vi "Trial data array-Initialise.vi"(6 "Total number of points in each \ntrial (or Z-plane), for both channels":u32, 8 "error in":errorcluster, 11 "Logging queue element":T1={"Imaging Protocol"=enum."Live Imaging", "Number of Trials"=0, "Frame Size"=512, "# Averaged frames"=0, "Dwell time (us)"=0.0, "Index of Z-plane"=0, "Timelapse?"=FALSE, "Logging process is active"=FALSE, "Speed logging enabled"=FALSE, "tdms file ref"=refnum, "path"=path "", "Trial Number"=0, "Expected # points acquired"=FALSE, "Manually stopped"=FALSE, "Last trial"=FALSE, "Ch0 data"=[], "Ch1 data"=[], "Ref Data"=[], "Ref Frame Time"=[], "Image Time"=[], "Continuous Time"=[], "Ref X Length"=0, "Ref Y Length"=0, "# Ref Averaged frames"=0, "Ref Dwell time (us)"=0.0, "Points acquired"={"Ch0 last trial"=0, "Ch1 last trial"=0, "All trials"=0}, "HW Timings File"=refnum} {"Ref Dwell time (us)" format="%#.6g"; "Frame Size" items=["100X100"=100, "128X128"=128, "200X200"=200, "256X256"=256, "512X512"=512, "1024x1024"=1024, "2048x2048"=2048]; "Dwell time (us)" format="%#.6g"}) -> (0 "error out":errorcluster, 1 "Initialised single trial or single plane data":dbl[](array[numeric]))   [LabVIEW 2020]
uses:
  Typedefs/Logging queue element.ctl
  Typedefs/Imaging Protocols enum.ctl
  Typedefs/Frame Size.ctl
  Typedefs/Acquired points count.ctl
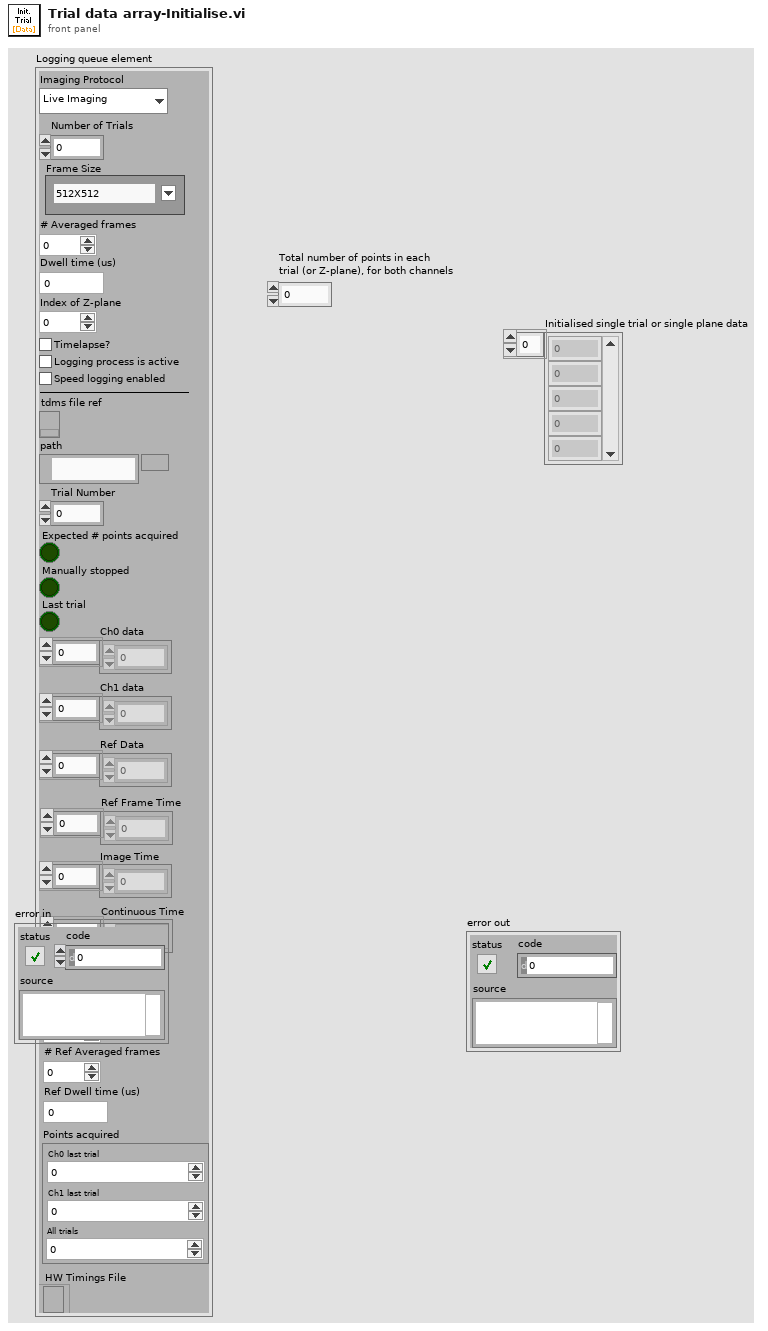
[diagram p1: front panel]
types:
  T1 = typedef "Logging queue element.ctl" = cluster{"Imaging Protocol":T2, "Number of Trials":u16, "Frame Size":T3, "# Averaged frames":u16, "Dwell time (us)":dbl, "Index of Z-plane":i32, "Timelapse?":bool, "Logging process is active":bool, "Speed logging enabled":bool, "tdms file ref":refnum<k34>, "path":path, "Trial Number":i32, "Expected # points acquired":bool, "Manually stopped":bool, "Last trial":bool, "Ch0 data":u32[], "Ch1 data":u32[], "Ref Data":u32[], "Ref Frame Time":u64[], "Image Time":u64[], "Continuous Time":u64[], "Ref X Length":u16, "Ref Y Length":u16, "# Ref Averaged frames":u16, "Ref Dwell time (us)":dbl, "Points acquired":T4, "HW Timings File":refnum<file>}
  T2 = typedef "Imaging Protocols enum.ctl" = enum16{"AOL Z-Stack", "Motor Z Stack", "Functional Acquisition", "Single Plane Acquisition", "Volume Acquisition", "Live Imaging", "Live Plane Imaging", "Live Volume Imaging"}
  T3 = typedef "Frame Size.ctl" = u16
  T4 = typedef "Acquired points count.ctl" = cluster{"Ch0 last trial":u64, "Ch1 last trial":u64, "All trials":u64}
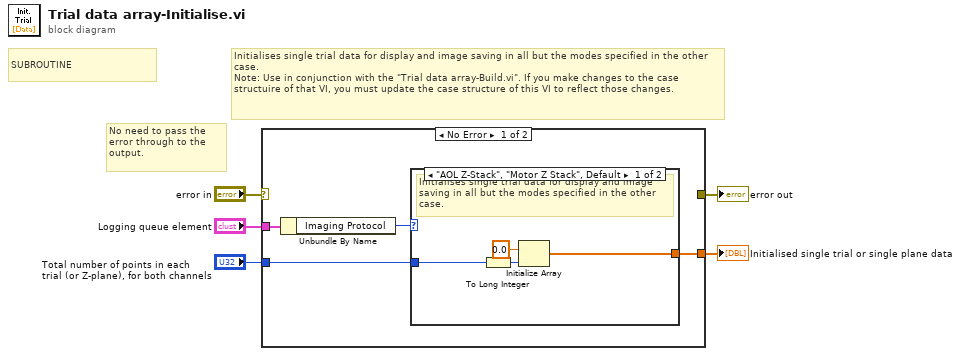
[diagram p0: block diagram]
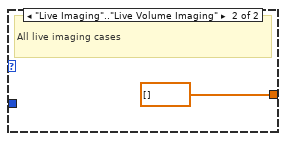
[diagram p2: hidden frame]
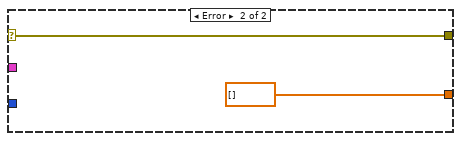
[diagram p3: hidden frame]
diagram:
  # "SUBROUTINE"
  # "Initialises single trial data for display and image saving in all but the modes specified in the other case.\nNote: Use in conjunction with the \"Trial data array-Build.vi\". If you make changes to the case structuire of that VI, you must update the case structure of this VI to reflect those changes."
  # "No need to pass the error through to the output."
  n1 = case shown="No Error" "error in" {
    selector: "error in" -> [_ w15]
    tunnel: "Logging queue element" -> [w9 _]
    tunnel: "Total number of points in each \ntrial (or Z-plane), for both channels" -> [w7 _]
    tunnel: [w6 dbl[] []] -> w2
    tunnel: [_ w15] -> w1
    frame No Error {
      n2 = Unbundle By Name(w9) -> ("Imaging Protocol"=w8:T2)
      n3 = case shown="\"AOL Z-Stack\", \"Motor Z Stack\", Default" w8 {
        tunnel: w7 -> [w11 _]
        tunnel: [w10 dbl[] []] -> w6
        frame "AOL Z-Stack", "Motor Z Stack", Default {
          # "Initialises single trial data for display and image saving in all but the modes specified in the other case."
          n4 = To Long Integer(number=w11) -> (32bit integer=w12:i32)
          n5 = Initialize Array(0.0, w12) -> (w10:dbl[])
        }
        frame "Live Imaging".."Live Volume Imaging" {
          # "All live imaging cases"
        }
      }
    }
    frame Error {
    }
  }
  "Initialised single trial or single plane data" <- w2
  "error out" <- w1
